vi "hextobcc.vi"(11 "输入校验十六进制":string) -> (0 "BCC校验结果":string)   [LabVIEW 2022 SP3]
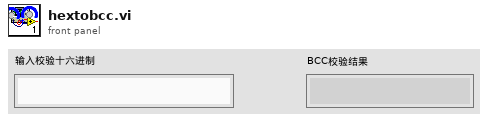
[diagram p1: front panel]
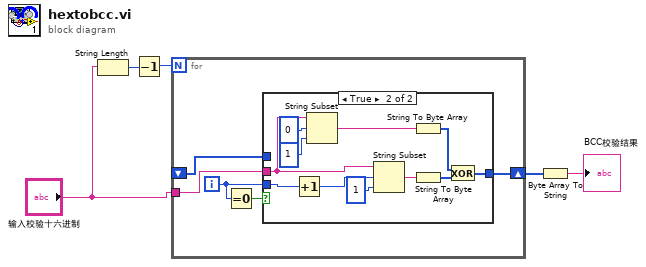
[diagram p0: block diagram]
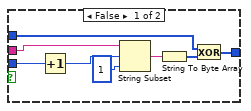
[diagram p2: hidden frame]
diagram:
  n1 = String Length(string="输入校验十六进制") -> (length=w5:i32)
  n2 = Decrement(x=w5) -> (x-1=w4:i32)
  n3 = for {
    N: w4 -> [_]
    tunnel: "输入校验十六进制" -> [w9]
    shift-right: [w6] -> w3
    shift-left: _ -> [w7]
    i -> [w8]
    n4 = Equal To 0?(x=w8) -> (x = 0?=w10:bool)
    n5 = case shown="True" w10 {
      tunnel: w9 -> [w18 w26]
      tunnel: w8 -> [w17 w24]
      tunnel: [w11 w19] -> w6
      tunnel: w7 -> [w13 _]
      frame False {
        n6 = Increment(x=w17) -> (x+1=w16:i32)
        n7 = String Subset(string=w18, offset (0)=w16, length (rest)=1 ("长度（剩余）")) -> (substring=w14:string)
        n8 = String To Byte Array(string=w14) -> (unsigned byte array=w12:u8[])
        n9 = Exclusive Or(1:w12, 2:w13) -> (0:w11:u8[])
      }
      frame True {
        n10 = Increment(x=w24) -> (x+1=w25:i32)
        n11 = String Subset(string=w26, offset (0)=0 ("偏移量(0)"), length (rest)=1 ("长度（剩余）")) -> (substring=w27:string)
        n12 = String Subset(string=w26, offset (0)=w25, length (rest)=1 ("长度（剩余）")) -> (substring=w22:string)
        n13 = String To Byte Array(string=w27) -> (unsigned byte array=w21:u8[])
        n14 = String To Byte Array(string=w22) -> (unsigned byte array=w20:u8[])
        n15 = Exclusive Or(1:w20, 2:w21) -> (0:w19:u8[])
      }
    }
  }
  n16 = Byte Array To String(unsigned byte array=w3) -> (string=→"BCC校验结果":string)
